vi "update Position coords.vi"(8 "error in (no error)":errorcluster, 10 "IK Parameters":T2, 11 "Data in":T1={"link 1 angle"=0.0, "link 2 angle"=0.0, "link 1 length"=0.0, "link 2 length"=0.0, "Current arm location"=[{"X"=0.0, "Y"=0.0}, {"X"=-37.249783598972314, "Y"=33.353464914904016}, {"X"=-74.49956719794463, "Y"=66.70692982980803}], "Link Picture"=bytes[1162], "Desired Location"={"Desired X"=0.0, "Desired Y"=0.0}, "Distance"=0.0, "Velocity (mm/s)"=0.0, "Next Location"={"Next X"=0.0, "Next Y"=0.0}, "Error"={"X error"=0.0, "Y error"=0.0}, "tdms data"=refnum}) -> (0 "error out":errorcluster, 3 "Data Out":T1={"link 1 angle"=0.0, "link 2 angle"=0.0, "link 1 length"=0.0, "link 2 length"=0.0, "Current arm location"=[{"X"=0.0, "Y"=0.0}, {"X"=-37.249783598972314, "Y"=33.353464914904016}, {"X"=-74.49956719794463, "Y"=66.70692982980803}], "Link Picture"=bytes[1162], "Desired Location"={"Desired X"=0.0, "Desired Y"=0.0}, "Distance"=0.0, "Velocity (mm/s)"=0.0, "Next Location"={"Next X"=0.0, "Next Y"=0.0}, "Error"={"X error"=0.0, "Y error"=0.0}, "tdms data"=refnum})   [LabVIEW 2016]
uses:
  Type Defs/IK parameters.ctl
  Type Defs/Host Data.ctl
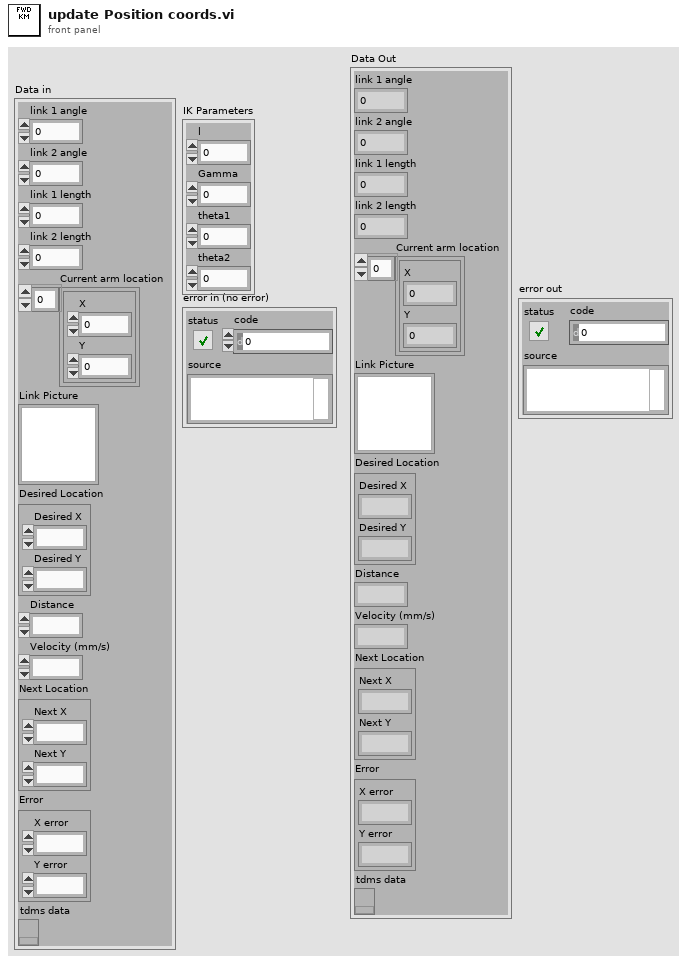
[diagram p1: front panel]
types:
  T1 = typedef "Host Data.ctl" = cluster{"link 1 angle":dbl, "link 2 angle":dbl, "link 1 length":dbl, "link 2 length":dbl, "Current arm location":cluster{"X":dbl, "Y":dbl}[], "Link Picture":picture, "Desired Location":cluster{"Desired X":dbl, "Desired Y":dbl}, "Distance":dbl, "Velocity (mm/s)":dbl, "Next Location":cluster{"Next X":dbl, "Next Y":dbl}, "Error":cluster{"X error":dbl, "Y error":dbl}, "tdms data":refnum<k34>}
  T2 = typedef "IK parameters.ctl" = cluster{"l":dbl, "Gamma":dbl, "theta1":dbl, "theta2":dbl}
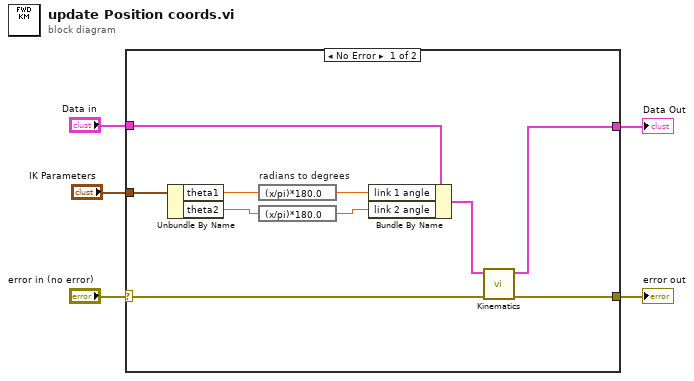
[diagram p0: block diagram]
diagram:
  n1 = case shown="No Error" "error in (no error)" {
    selector: "error in (no error)" -> [w13 w17]
    tunnel: [w12 w17] -> w4
    tunnel: "Data in" -> [w15 w16]
    tunnel: "IK Parameters" -> [w14 _]
    tunnel: [w10 w16] -> w1
    frame No Error {
      n2 = Unbundle By Name(w14) -> ("theta1"=w9:dbl, "theta2"=w7:dbl)
      n3 = expression code="(x/pi)*180.0" "radians to degrees"(w9) -> (w8:dbl)
      n4 = expression code="(x/pi)*180.0" ("radians to degrees")(w7) -> (w6:dbl)
      n5 = Bundle By Name(cluster=w15, "link 1 angle"=w8, "link 2 angle"=w6) -> (w11:T1)
      n6 = call "Kinematics.vi"("error in (no error)"=w13, "Data In"=w11) -> ("error out"=w12:errorcluster, "Data Out"=w10:T1)  [unwired: 8 in]
    }
    frame Error {
    }
  }
  "error out" <- w4
  "Data Out" <- w1
